vi "Destroy Registry.vi"(8 "error in (no error)":errorcluster, 11 "Registry in":refnum<data-value>) -> (0 "error out":errorcluster, 2 "Remaining Nodes":refnum<class "UniqueName.lvclass">[](array[class]))   [LabVIEW 2014, in "UniqueName.lvlib" / "NameRegistry.lvclass"]
uses:
  NameRegistry.lvclass
  UniqueNameClass/UniqueName.lvclass
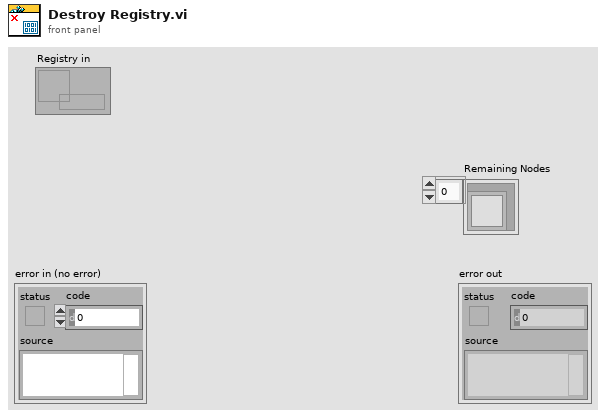
[diagram p1: front panel]
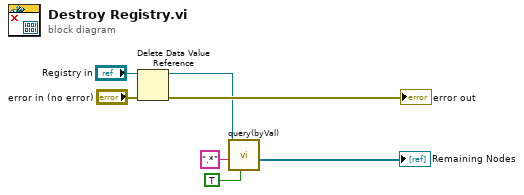
[diagram p0: block diagram]
diagram:
  n1 = Delete Data Value Reference(data value reference="Registry in", error in="error in (no error)") -> (data value=w4:refnum<class "NameRegistry.lvclass">, error out=→"error out":errorcluster)
  n2 = call "query(byVal).vi"("use Regex? (F)"=TRUE, "Search string"=".*", "Instance"=w4) -> ("Nodes"=→"Remaining Nodes":refnum<class "UniqueName.lvclass">[])  [unwired: 5 in, 3 out]
